vi "BlankRunningVI.vi"   [LabVIEW 2023]
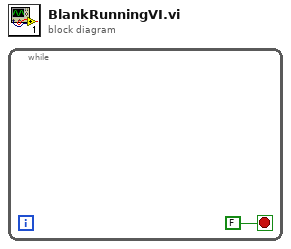
[diagram p0: block diagram]
diagram:
  n1 = while {
    stop <- FALSE stop-if-true
  }
